vi "LabVIEW-Arduino C Code-Gen.vi"() -> ()   [LabVIEW 2014]
uses:
  <vilib>/Aledyne-TSXperts/Arduino Compatible Compiler for LabVIEW/Code Generator/Compilation/CompileOptions.ctl
  <vilib>/Aledyne-TSXperts/Arduino Compatible Compiler for LabVIEW/Code Generator/Compilation/Compilation Type.ctl
  <vilib>/Aledyne-TSXperts/Arduino Compatible Compiler for LabVIEW/Code Generator/Compilation/Board Identifier.ctl
  <vilib>/Aledyne-TSXperts/Arduino Compatible Compiler for LabVIEW/Arduino Compatible Compiler for LabVIEW.lvlib
panel:
  out "Sketch":string
  out "Compile Error":bool
  out "Status Output":string
  out "SketchPath":path
  in  "board":T1={"Display Name"="WeMos D1 (LabVIEW)", "Architecture"="esp8266", "Board"="d1", "cpu"=[], "SelectedCPU"="", "package"="qwavesys"}
  in  "Delete Sketch After Build":bool
  in  "Port":string="COM4"
  in  "Compilation Type":T2
  in  "CompileOptions":T3
  in  "VIPath":path
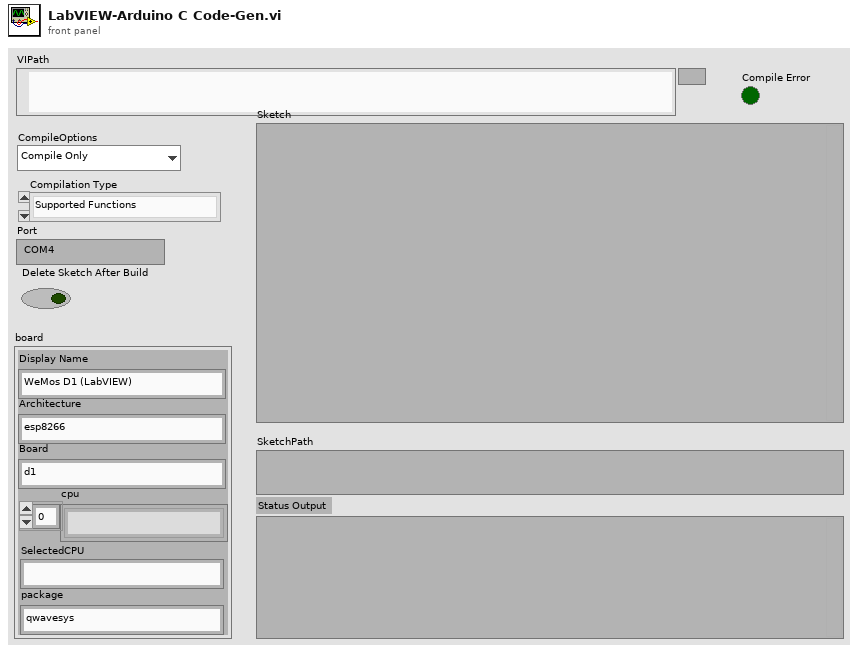
[diagram p1: front panel]
types:
  T1 = typedef "Arduino Compatible Compiler for LabVIEW.lvlib/Board Identifier.ctl" = cluster{"Display Name":string, "Architecture":string, "Board":string, "cpu":string[], "SelectedCPU":string, "package":string}
  T2 = typedef "Arduino Compatible Compiler for LabVIEW.lvlib/Compilation Type.ctl" = enum16{"Supported Functions", "User Library"}
  T3 = typedef "Arduino Compatible Compiler for LabVIEW.lvlib/CompileOptions.ctl" = enum16{"Compile Only", "Compile And Download", "Doesn't Compile"}
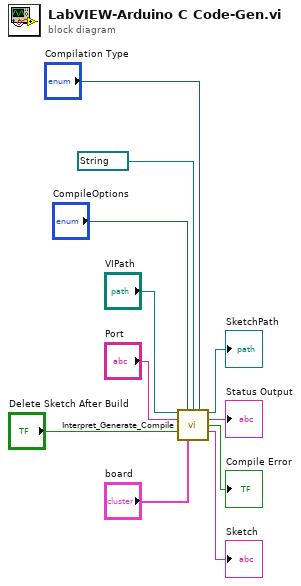
[diagram p0: block diagram]
diagram:
  n1 = call <vilib>:"Interpret_Generate_Compile.vi"("VIPath"="VIPath", "CompileOptions"="CompileOptions", "Status"=refnum<vi> refnum, "Compilation Type"="Compilation Type", "Port"="Port", "Delete Sketch After Build"="Delete Sketch After Build", "board"="board") -> ("SketchPath"=→"SketchPath":path, "Status Output"=→"Status Output":string, "Compile Error"=→"Compile Error":bool, "Sketch"=→"Sketch":string)  [unwired: 4 in, 1 out]
